vi "Match first tags ASCII and Unicode V2.vi"(6 "Type and run direction":T1=enum."ASCII", 9 "Hyperlink":string, 11 "Text":string) -> (1 "Array":T3(array[cluster]), 3 "Find tag ?":bool)   [LabVIEW 2019]
doc: "Version 2.0\nDeveloped by Jean-Marc Simard\nCopyright © 2010, Exaprom Inc.\nAll rights reserved.\nLicense: BSD"
uses:
  <userlib>/Exaprom PDF/Controls/Text Controls/Text type.ctl
  <userlib>/Exaprom PDF/Controls/Text Controls/Unicode/Type and run direction.ctl
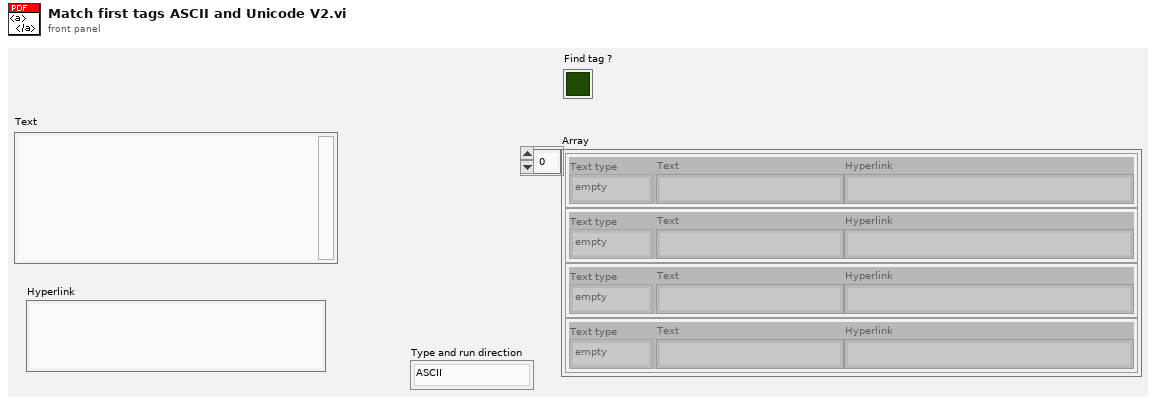
[diagram p1: front panel]
types:
  T1 = typedef "Type and run direction.ctl" = enum16{"Select", "ASCII", "UTF-16", "UTF-16 (default)", "UTF-16 (LTR)", "UTF-16 (RTL)"}
  T2 = typedef "Text type.ctl" = enum16{"empty", "Text", "Hyperlink"}
  T3 = cluster{"Text type":T2, "Text":string, "Hyperlink":string}[]
  T4 = cluster{"Text type":T2, "Text type":T2, "Text type":T2}
  T5 = cluster{"Text type":T2, "Text":string, "Hyperlink":string}
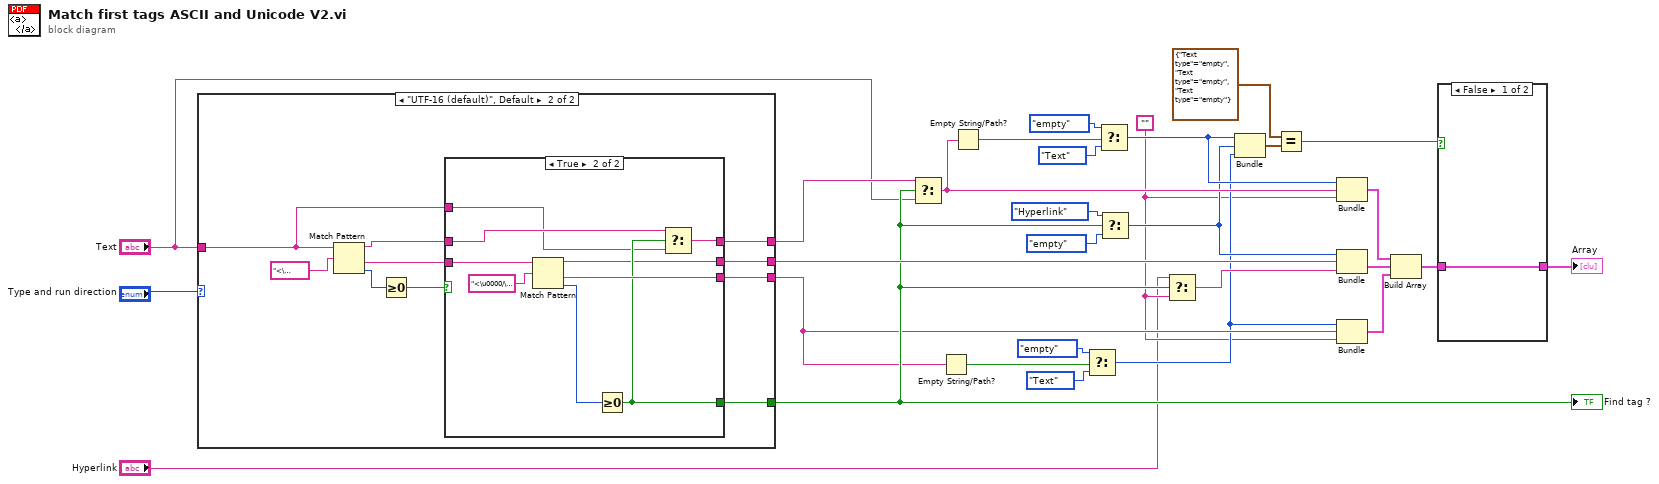
[diagram p0: block diagram]
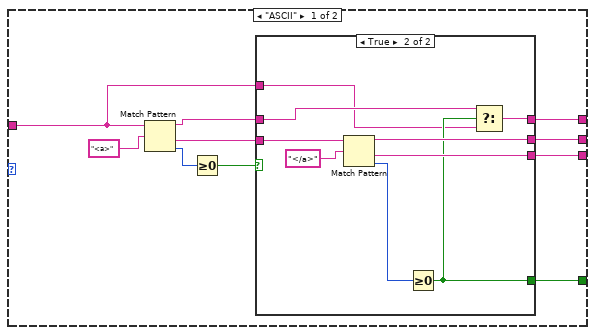
[diagram p2: hidden frame]
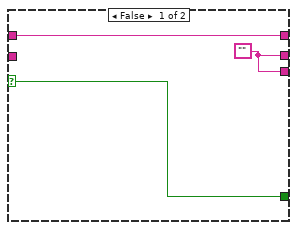
[diagram p3: hidden frame]
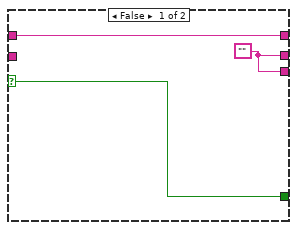
[diagram p4: hidden frame]
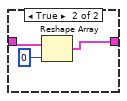
[diagram p5: hidden frame]
diagram:
  w4 = ""
  n1 = case shown="\"UTF-16 (default)\", Default" "Type and run direction" {
    tunnel: [w34 w56] -> w29
    tunnel: [w33 w55] -> w24
    tunnel: [w32 w54] -> w18
    tunnel: [w31 w53] -> w13
    tunnel: "Text" -> [w30 w52]
    frame "ASCII" {
      n2 = Match Pattern(string=w30, regular expression="<a>") -> (before substring=w36:string, after substring=w35:string, offset past match=w39:i32)  [unwired: 2 out]
      n3 = Greater Or Equal To 0?(x=w39) -> (x >= 0?=w38:bool)
      n4 = case shown="True" w38 {
        selector: w38 -> [w40 _]
        tunnel: w36 -> [w42 w44]
        tunnel: [w42 w46] -> w33
        tunnel: w35 -> [_ w51]
        tunnel: [w41 w49] -> w34
        tunnel: [w41 w48] -> w31
        tunnel: [w40 w45] -> w32
        tunnel: w30 -> [_ w43]
        frame False {
          w41 = ""
        }
        frame True {
          n5 = Match Pattern(string=w51, regular expression="</a>") -> (before substring=w49:string, after substring=w48:string, offset past match=w47:i32)  [unwired: 2 out]
          n6 = Greater Or Equal To 0?(x=w47) -> (x >= 0?=w45:bool)
          n7 = Select(t=w44, s=w45, f=w43) -> (s? t:f=w46:string)
        }
      }
    }
    frame "UTF-16 (default)", Default {
      n8 = Match Pattern(string=w52, regular expression="<\u0000a\u0000>\u0000") -> (before substring=w58:string, after substring=w57:string, offset past match=w61:i32)  [unwired: 2 out]
      n9 = Greater Or Equal To 0?(x=w61) -> (x >= 0?=w60:bool)
      n10 = case shown="True" w60 {
        selector: w60 -> [w62 _]
        tunnel: w58 -> [w64 w67]
        tunnel: [w64 w69] -> w55
        tunnel: w57 -> [_ w73]
        tunnel: [w63 w65] -> w56
        tunnel: [w63 w71] -> w53
        tunnel: [w62 w68] -> w54
        tunnel: w52 -> [_ w66]
        frame False {
          w63 = ""
        }
        frame True {
          n11 = Match Pattern(string=w73, regular expression="<\u0000/\u0000a\u0000>\u0000") -> (before substring=w65:string, after substring=w71:string, offset past match=w70:i32)  [unwired: 2 out]
          n12 = Greater Or Equal To 0?(x=w70) -> (x >= 0?=w68:bool)
          n13 = Select(t=w67, s=w68, f=w66) -> (s? t:f=w69:string)
        }
      }
    }
  }
  "Find tag ?" <- w18
  n14 = Select(t=w24, s=w18, f="Text") -> (s? t:f=w17:string)
  n15 = Empty String/Path?(string/path=w13) -> (empty?=w14:bool)
  n16 = Empty String/Path?(string/path=w17) -> (empty?=w23:bool)
  n17 = Select(t=Text_type."empty" ("Text type"), s=w14, f=Text_type."Text" ("Text type")) -> (s? t:f=w10:T2)
  n18 = Select(t=Text_type."empty" ("Text type"), s=w23, f=Text_type."Text" ("Text type")) -> (s? t:f=w12:T2)
  n19 = Select(t=Text_type."Hyperlink" ("Text type"), s=w18, f=Text_type."empty" ("Text type")) -> (s? t:f=w11:T2)
  n20 = Select(t="Hyperlink", s=w18, f=w4) -> (s? t:f=w28:string)
  n21 = Bundle("Text type"=w12, "Text type"=w11, "Text type"=w10) -> (w9:T4)  [unwired: 1 out]
  n22 = Equal?(x=T4 {"Text type"=enum."empty", "Text type"=enum."empty", "Text type"=enum."empty"}, y=w9) -> (x = y?=w7:bool)
  n23 = Bundle("Text type"=w12, "Text"=w17, w4) -> (w27:cluster{"Text type":T2, "Text":string, string})  [unwired: 1 out]
  n24 = Bundle("Text type"=w11, "Text"=w29, "Hyperlink"=w28) -> (w26:T5)  [unwired: 1 out]
  n25 = Bundle("Text type"=w10, "Text"=w13, w4) -> (w25:cluster{"Text type":T2, "Text":string, string})  [unwired: 1 out]
  n26 = Build Array(w27, w26, w25) -> (w6:T3)
  n27 = case shown="False" w7 {
    tunnel: w6 -> [w74 w77]
    tunnel: [w74 w76] -> w5
    frame False {
    }
    frame True {
      n28 = Reshape Array(w77, 0 ("dimension size")) -> (w76:T3)
    }
  }
  "Array" <- w5
